vi "Task Init.vi"(8 "error in (no error)":errorcluster, 11 "DebugGUI in":refnum<class "DebugGUI.lvclass">) -> (0 "error out":errorcluster, 3 "DebugGUI out":refnum<class "DebugGUI.lvclass">)   [LabVIEW 2020, in "Volatus.lvlib" / "DebugGUI.lvclass"]
uses:
  DebugGUI.lvclass
  DebugGUI.lvclass/DebugGUI.ctl
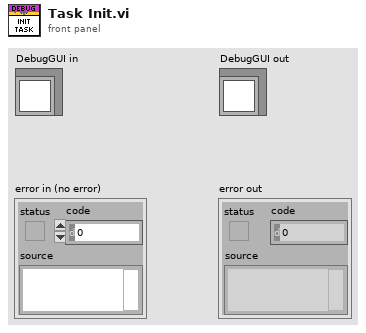
[diagram p1: front panel]
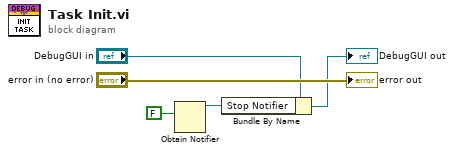
[diagram p0: block diagram]
diagram:
  n1 = Obtain Notifier(notification data type=FALSE) -> (notifier out=w3:refnum<notifier>)  [unwired: 3 in, 2 out]
  n2 = Bundle By Name(cluster="DebugGUI in", "Stop Notifier"=w3) -> (→"DebugGUI out":refnum<class "DebugGUI.lvclass">)
  "error out" <- "error in (no error)"
